vi "Bind RPC ni_measurements_v1_MeasurementService_GetMetadata.vi"(11 "gRPCid server in":T3) -> (0 "error out":errorcluster, 1 "ni_measurements_v1_MeasurementService_GetMetadata Internal UE":T2, 2 "ni_measurements_v1_MeasurementService_GetMetadata gRPC UE":T1, 3 "gRPCid server out":T3)   [LabVIEW 2020, in "LineRegulation.lvlib" / "MeasurementService.lvclass"]
uses:
  MeasurementService.lvclass
  <vilib>/gRPC/LabVIEW gRPC Library/Server API/typeDefs/grpcId.ctl
  typeDefs/Server Internal Message UE.ctl
  typeDefs/Server Internal Message.ctl
  <vilib>/gRPC/LabVIEW gRPC Library/Server API/typeDefs/gRPCId Cluster UE.ctl
  <vilib>/gRPC/LabVIEW gRPC Library/Server API/typeDefs/gRPCId Cluster.ctl
  616620f9-6bbe-466a-af51-04bcc3596ea0.vi
  <vilib>/gRPC/LabVIEW gRPC Library/Server API/Server/Get Server DLL Path.vi
  MeasurementService.lvclass/MeasurementService.ctl
  <vilib>/gRPC/LabVIEW gRPC Library/gprc-lvsupport-release.lvlib
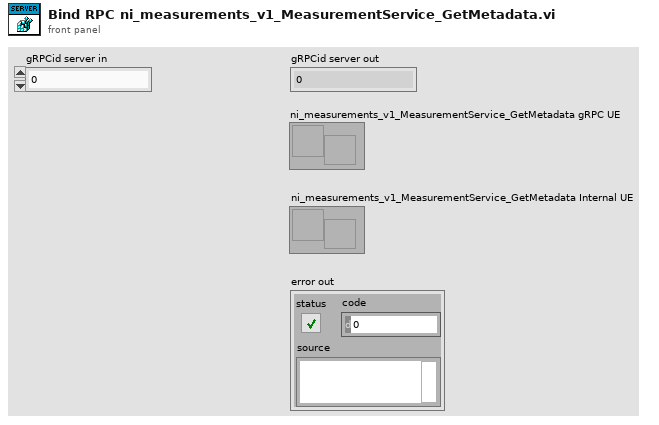
[diagram p1: front panel]
types:
  T1 = typedef "gprc-lvsupport-release.lvlib/gRPCId Cluster UE.ctl" = refnum<user-event>
  T2 = typedef "LineRegulation.lvlib/MeasurementService.lvclass/Server Internal Message UE.ctl" = refnum<user-event>
  T3 = typedef "gprc-lvsupport-release.lvlib/grpcId.ctl" = u64
  T4 = typedef "LineRegulation.lvlib/MeasurementService.lvclass/Server Internal Message.ctl" = cluster{"Command":string, "Data":variant}
  T5 = typedef "gprc-lvsupport-release.lvlib/gRPCId Cluster.ctl" = cluster{"gRPCid":T3}
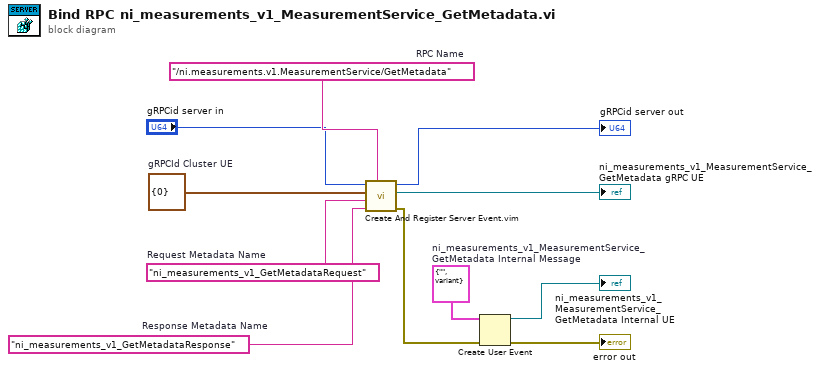
[diagram p0: block diagram]
diagram:
  w5 = T4 {"Command"="", "Data"=variant}  # ni_measurements_v1_MeasurementService_GetMetadata Internal Message
  w8 = "ni_measurements_v1_GetMetadataResponse"  # Response Metadata Name
  w11 = T5 {"gRPCid"=0}  # gRPCId Cluster UE
  w9 = "ni_measurements_v1_GetMetadataRequest"  # Request Metadata Name
  w10 = "/ni.measurements.v1.MeasurementService/GetMetadata"  # RPC Name
  n1 = call "Create And Register Server Event.vim"("Method name"=w10, "Response Metadata Name"=w8, "Request Metadata Name"=w9, "event in"=w11, "gRPCid server in"="gRPCid server in") -> ("error out"=w4:errorcluster, "event"=→"ni_measurements_v1_MeasurementService_GetMetadata gRPC UE":refnum<user-event>, "gRPCid server out"=→"gRPCid server out":T3)  [unwired: 4 in]
  n2 = Create User Event(user event datatype=w5, error in=w4) -> (user event=→"ni_measurements_v1_MeasurementService_GetMetadata Internal UE":refnum<user-event>, error out=→"error out":errorcluster)
